vi "OAT Orbit Plot (Unfiltered).vi"(0 "even-angle signals":cluster{"r0":dbl, "dr":dbl, "Y":dbl[]}[](array[cluster]) {"r0" format="%.2p"; "dr" format="%.2p"; "Y" format="%.2f"}, 1 "orbit plot ref":refnum<vi>, 2 "reset? (F)":bool, 5 "speed profile":T1 {"speed [RPM]" format="%.2f"; "time [s]" format="%.2f"}, 7 "even-angle position info":T3, 9 "revolutions to display [rev]":cluster{"start":dbl, "duration":dbl}={"start"=0.0, "duration"=1.0} {"duration" format="%.2f"; "start" format="%.2f"}, 11 "error in (no error)":errorcluster, 12 "channel settings":T2={"shaft rotating direction"=0, "probe angles [deg]"={"X"=0, "Y"=90}} {"probe angles [deg]"."Y" max=360 step=1; "probe angles [deg]"."X" max=360 step=1; "shaft rotating direction" items=["CCW", "CW"]}) -> (4 "orbit plot":T4, 15 "error out":errorcluster)   [LabVIEW 2017]
doc: "Draws an orbit plot with unfiltered or filtered data on an XY graph. The unfiltered data comes from the <B>even-angle signals</B> input, and the filtered data comes from the <B>magnitudes</B> and <B>phases [phase lag]</B> inputs."
uses:
  <vilib>/addons/Sound and Vibration/Order Analysis/Backward Compatibility/SubVIs/oa_Orbit Plot Control.ctl
  <vilib>/addons/Sound and Vibration/Order Analysis/Misc/OAT Position Info.ctl
  <vilib>/addons/Sound and Vibration/Order Analysis/Tach Process/SubVIs/speed profile.ctl
  <vilib>/addons/Sound and Vibration/Order Analysis/Resample Order Tracking/SoundVib_Resampling.lvlib
  <vilib>/addons/Sound and Vibration/Order Analysis/Tach Process/SoundVib_TachProcess.lvlib
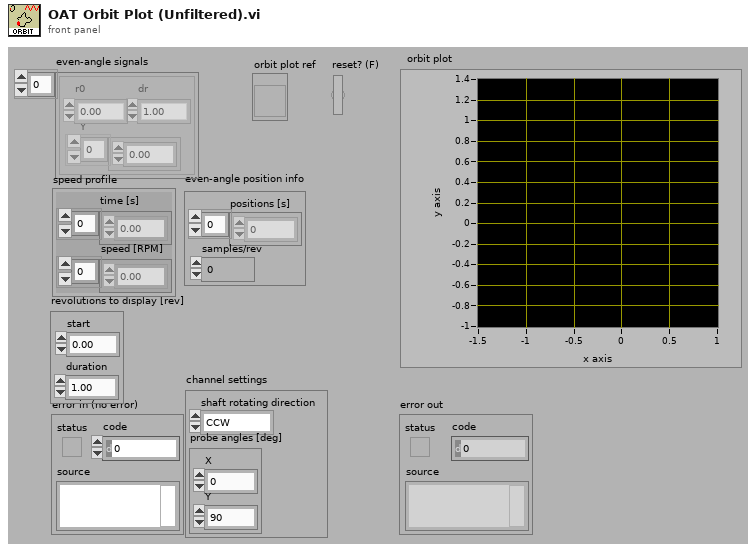
[diagram p1: front panel]
types:
  T1 = typedef "SoundVib_TachProcess.lvlib/speed profile.ctl" = cluster{"time [s]":dbl[], "speed [RPM]":dbl[]}
  T2 = cluster{"shaft rotating direction":u16, "probe angles [deg]":cluster{"X":u32, "Y":u32}}
  T3 = typedef "OAT Position Info.ctl" = cluster{"positions [s]":dbl[], "samples/rev":dbl}
  T4 = typedef "oa_Orbit Plot Control.ctl" = cluster{dbl[], dbl[]}[]
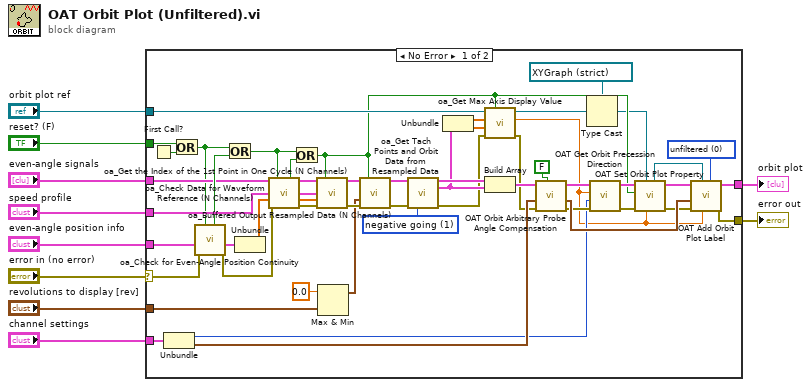
[diagram p0: block diagram]
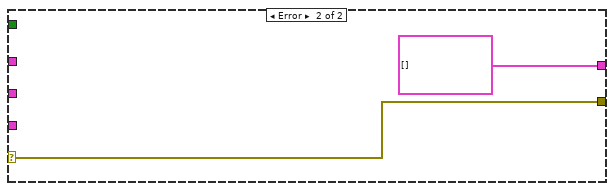
[diagram p2: hidden frame]
diagram:
  n1 = case shown="No Error" "error in (no error)" {
    selector: "error in (no error)" -> [w19 w65]
    tunnel: [w35 w65] -> w9
    tunnel: "even-angle signals" -> [w17 _]
    tunnel: "speed profile" -> [w59 _]
    tunnel: "even-angle position info" -> [w16 _]
    tunnel: "reset? (F)" -> [w22 _]
    tunnel: "revolutions to display [rev]" -> [w56 _]
    tunnel: [w46 cluster{dbl[], dbl[]}[] [] ("XY plot data out")] -> w4
    tunnel: "channel settings" -> [w45 _]
    tunnel: "orbit plot ref" -> [w30 _]
    frame No Error {
      w31 = u16 1 items=["positive going", "negative going"] ("trigger pulse direction")
      w47 = u16 0 items=["unfiltered", "filtered"] ("plot type")
      n2 = First Call?() -> (First Call?: T/F=w23:bool)
      n3 = Unbundle(w45) -> ("shaft rotating direction"=w38:u16, "probe angles [deg]"=w44:cluster{"X":u32, "Y":u32})
      n4 = Or(x=w22, y=w23) -> (x .or. y?=w14:bool)
      n5 = call <vilib>:"oa_Check for Even-Angle Position Continuity.vi"("reset in"=w14, "error in (no error)"=w19, "even-angle position info"=w16) -> ("error out"=w18:errorcluster, "even-angle position info dup"=w15:T3, "position not continuous"=w21:bool)  [unwired: 6 in]
      n6 = Or(x=w14, y=w21) -> (x .or. y?=w20:bool)
      n7 = Unbundle(w15) -> ("positions [s]"=w34:dbl[])  [unwired: 1 out]
      n8 = call <vilib>:"oa_Check Data for Waveform Reference (N Channels).vi"("resampled signal"=w17, "reset? (True)"=w20, "speed profile"=w59, "interpolated pulse positions"=w34, "error in (no error)"=w18) -> ("reset"=w58:bool, "resampled data out"=w62:cluster{"r0":dbl, "dr":dbl, "Y":dbl[]}[], "speed profile out"=w60:T1, "interpolated pulse positions out"=w61:dbl[], "error out"=w63:errorcluster)  [unwired: 3 in, 3 out]
      n9 = Or(x=w20, y=w58) -> (x .or. y?=w24:bool)
      n10 = call <vilib>:"oa_Get the Index of the 1st Point in One Cycle (N Channels).vi"("resampled signal"=w62, "reset? (True)"=w24, "speed profile"=w60, "interpolated pulse positions"=w61, "error in (no error)"=w63) -> ("resampled signal out"=w57:cluster{"r0":dbl, "dr":dbl, "Y":dbl[]}[], "error out"=w55:errorcluster)  [unwired: 8 in, 1 out]
      n11 = Max & Min(x=0.0, y=w56) -> (max(x,y)=w32:cluster{"start":dbl, "duration":dbl})  [unwired: 1 out]
      n12 = call <vilib>:"oa_Buffered Output Resampled Data (N Channels).vi"("resampled signal in"=w57, "reset? (True)"=w24, "display revolutions"=w32, "error in"=w55) -> ("resampled signal out"=w43:cluster{"r0":dbl, "dr":dbl, "Y":dbl[]}[], "error out"=w42:errorcluster)  [unwired: 9 in, 1 out]
      n13 = call <vilib>:"oa_Get Tach Points and Orbit Data from Resampled Data.vi"("resampled signal in"=w43, "error in"=w42, "trigger pulse direction"=w31) -> ("tach points"=w41:cluster{dbl[], dbl[]}, "orbit"=w40:cluster{dbl[], dbl[]}, "error out"=w29:errorcluster)  [unwired: 10 in]
      n14 = Unbundle(w40) -> (w26:dbl[], w25:dbl[])
      n15 = call <vilib>:"oa_Get Max Axis Display Value.vi"("reset? (F)"=w24, "error in (no error)"=w29, "orbit data Y"=w25, "orbit data X"=w26, "orbit plot ref"=w30) -> ("error out"=w28:errorcluster, "max data value out"=w27:dbl, "orbit plot out"=w12:refnum<vi>)  [unwired: 4 in]
      n16 = Build Array(w41, w40) -> (w50:cluster{dbl[], dbl[]}[])
      n17 = call <vilib>:"OAT Orbit Arbitrary Probe Angle Compensation.vi"("select methods"=FALSE, "error in (no error)"=w28, "probe angle"=w44, "XY plot data in"=w50) -> ("error out"=w39:errorcluster, "probe angle out"=w49:cluster{"X (red)":dbl, "Y (blue)":dbl}, "XY plot data out"=w54:cluster{dbl[], dbl[]}[])  [unwired: 5 in]
      n18 = Type Cast(type=refnum<vi> refnum ("orbit plot ref"), x=w12) -> (*(type *) &x=w11:refnum<vi>)
      n19 = call <vilib>:"OAT Get Orbit Precession Direction.vi"("error in (no error)"=w39, "shaft rotating direction"=w38, "max data value"=w27, "XY plot data in"=w54) -> ("error out"=w37:errorcluster, "XY plot data out"=w53:cluster{dbl[], dbl[]}[])  [unwired: 6 in]
      n20 = call <vilib>:"OAT Set Orbit Plot Property.vi"("max value"=w27, "orbit plot ref"=w11, "error in (no error)"=w37, "reset? (F)"=w24, "XY plot data in"=w53) -> ("error out"=w36:errorcluster, "XY plot data out"=w52:cluster{dbl[], dbl[]}[], "orbit plot ref"=w51:refnum<vi>)  [unwired: 4 in]
      n21 = call <vilib>:"OAT Add Orbit Plot Label.vi"("plot type"=w47, "max value"=w27, "orbit plot ref"=w51, "error in (no error)"=w36, "probe angle out"=w49, "XY plot data in"=w52) -> ("error out"=w35:errorcluster, "XY plot data out"=w46:cluster{dbl[], dbl[]}[])  [unwired: 4 in]
    }
    frame Error {
    }
  }
  "orbit plot" <- w4
  "error out" <- w9
